vi "ReadPluginINIFilePathRequest.vi"(8 "error in (no error)":errorcluster, 11 "ModuleID":i32=-1) -> (0 "error out":errorcluster)   [LabVIEW 2014, in "FlagImpairModule.lvlib"]
uses:
  FlagImpairModule.lvlib
  clEventType.ctl
  <vilib>/Utility/error.llb/Error Cluster From Error Code.vi
  <vilib>/ErrorRing/Error Ring.xnode
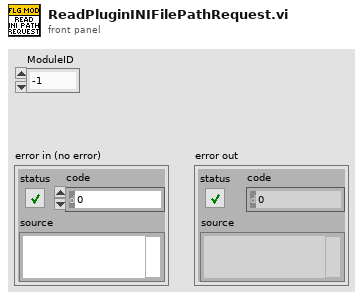
[diagram p1: front panel]
types:
  T1 = typedef "FlagImpairModule.lvlib/clRequestEvents.ctl" = cluster{"StopRequest":refnum<user-event>, "WriteFlagImpairConfigRequest":refnum<user-event>, "ReadFlagImpairConfigRequest":refnum<user-event>, "WriteFlagImpairParamsRequest":refnum<user-event>, "ReadFlagImpairParamsRequest":refnum<user-event>, "WriteTimeArrayRequest":refnum<user-event>, "ReadTimeArrayRequest":refnum<user-event>, "GetFlagImpairmentRequest":refnum<user-event>, "LoadPluginRequest":refnum<user-event>, "ReadPluginPathRequest":refnum<user-event>, "ShowPanelRequest":refnum<user-event>}
  T2 = typedef "FlagImpairModule.lvlib/clEventType.ctl" = cluster{"ModuleID":i32, "Data":variant}
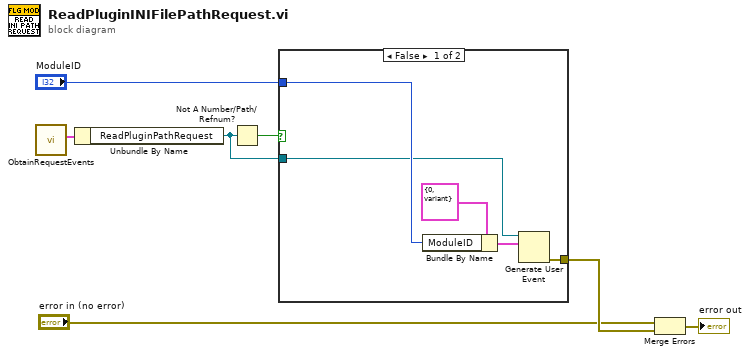
[diagram p0: block diagram]
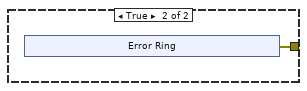
[diagram p2: hidden frame]
diagram:
  n1 = call "ObtainRequestEvents.vi"() -> ("clRequestEvents"=w7:T1)  [unwired: 10 in, 1 out]
  n2 = Unbundle By Name(w7) -> ("ReadPluginPathRequest"=w5:refnum<user-event>)
  n3 = Not A Number/Path/Refnum?(number/path/refnum=w5) -> (NaN/Path/Refnum?=w6:bool)
  n4 = case shown="False" w6 {
    tunnel: w5 -> [w10 _]
    tunnel: "ModuleID" -> [w11 _]
    tunnel: [w8 w13] -> w2
    frame False {
      n5 = Bundle By Name(cluster=T2 {"ModuleID"=0, "Data"=variant} ("clEventType"), "ModuleID"=w11) -> (w9:T2)
      n6 = Generate User Event(user event=w10, event data cluster=w9) -> (error out=w8:errorcluster)  [unwired: 2 in, 1 out]
    }
    frame True {
      n7 = xnode "Error Ring"() -> ("error out"=w13:errorcluster)
    }
  }
  n8 = Merge Errors("error in (no error)", w2) -> (→"error out":errorcluster)
